vi "variantCtrlNumericRegister.vi"(6 "menu":enum16{"get", "set"}(ring), 8 "error in":errorcluster, 9 "procNumericRegister in":dbl, 11 "procElement":variant) -> (0 "error out":errorcluster, 1 "procNumericRegister out":dbl, 3 "procElement out":variant)   [LabVIEW 2024]
uses:
  controls/typeProcVarientName.ctl
  variantCtrlNumber.vi
  proc.util.validateParamExist.vi
  <vilib>/Utility/error.llb/Clear Errors.vi
  util.error.create.vi
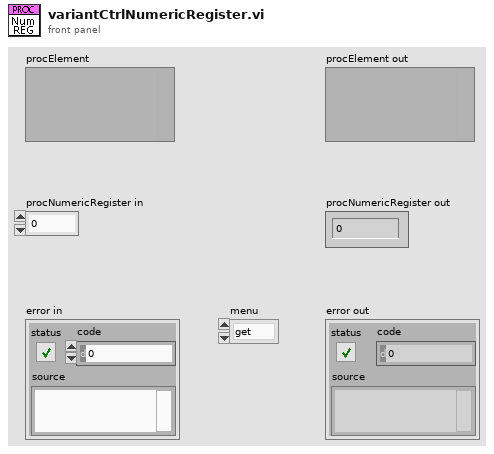
[diagram p1: front panel]
types:
  T1 = typedef "typeProcVarientName.ctl" = enum16{"procNameID", "procModuleID", "procPath", "procIsRunning", "procIndex", "procModule", "procRegisterNumeric", "procRegisterString", "procReport", "procReportPrev", "procCLK", "procStepPointer", "procType"}
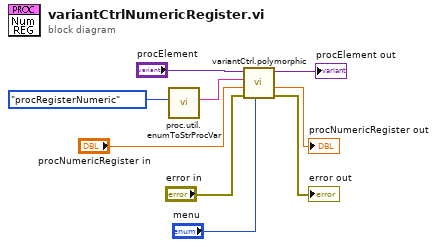
[diagram p0: block diagram]
diagram:
  n1 = call "proc.util.enumToStrProcVar.vi"("Proc var"=typeProcVarientName."procRegisterNumeric" ("proc var")) -> ("String"=w4:string)  [unwired: 10 in]
  n2 = call-poly "variantCtrl.polymorphic.vi"("menu in (get)"="menu", "error in"="error in", "number"="procNumericRegister in", "name in"=w4, "variant in"="procElement") -> ("error out"=→"error out":errorcluster, "number"=→"procNumericRegister out":dbl, "variant out"=→"procElement out":variant)  [unwired: 3 in, 1 out]
